vi "Subtract background.vi"(4 "Bin":dbl=0.05, 6 "Smoothing":dbl=32.0 format="%0.4f", 10 "Background":path=path "C:/Data/February_2015/021015/PDO_perp/s024_021015_TDO001.dat", 11 "Data":path=path "C:/Data/February_2015/021015/PDO_perp/s007_021015_TDO001.dat") -> (3 "XY Graph":cluster{"Output":dbl[], dbl[]}[](graph))   [LabVIEW 2018]
uses:
  <vilib>/Analysis/polynomials.llb/1D Polynomial Evaluation (DBL).vi
  <vilib>/Utility/file.llb/Write To Spreadsheet File (DBL).vi
  <vilib>/Analysis/NI_AALPro.lvlib
panel:
  in  "Keep old data":bool
  in  "Save result":bool=TRUE
  out "Waveform Graph":dbl[][](graph)
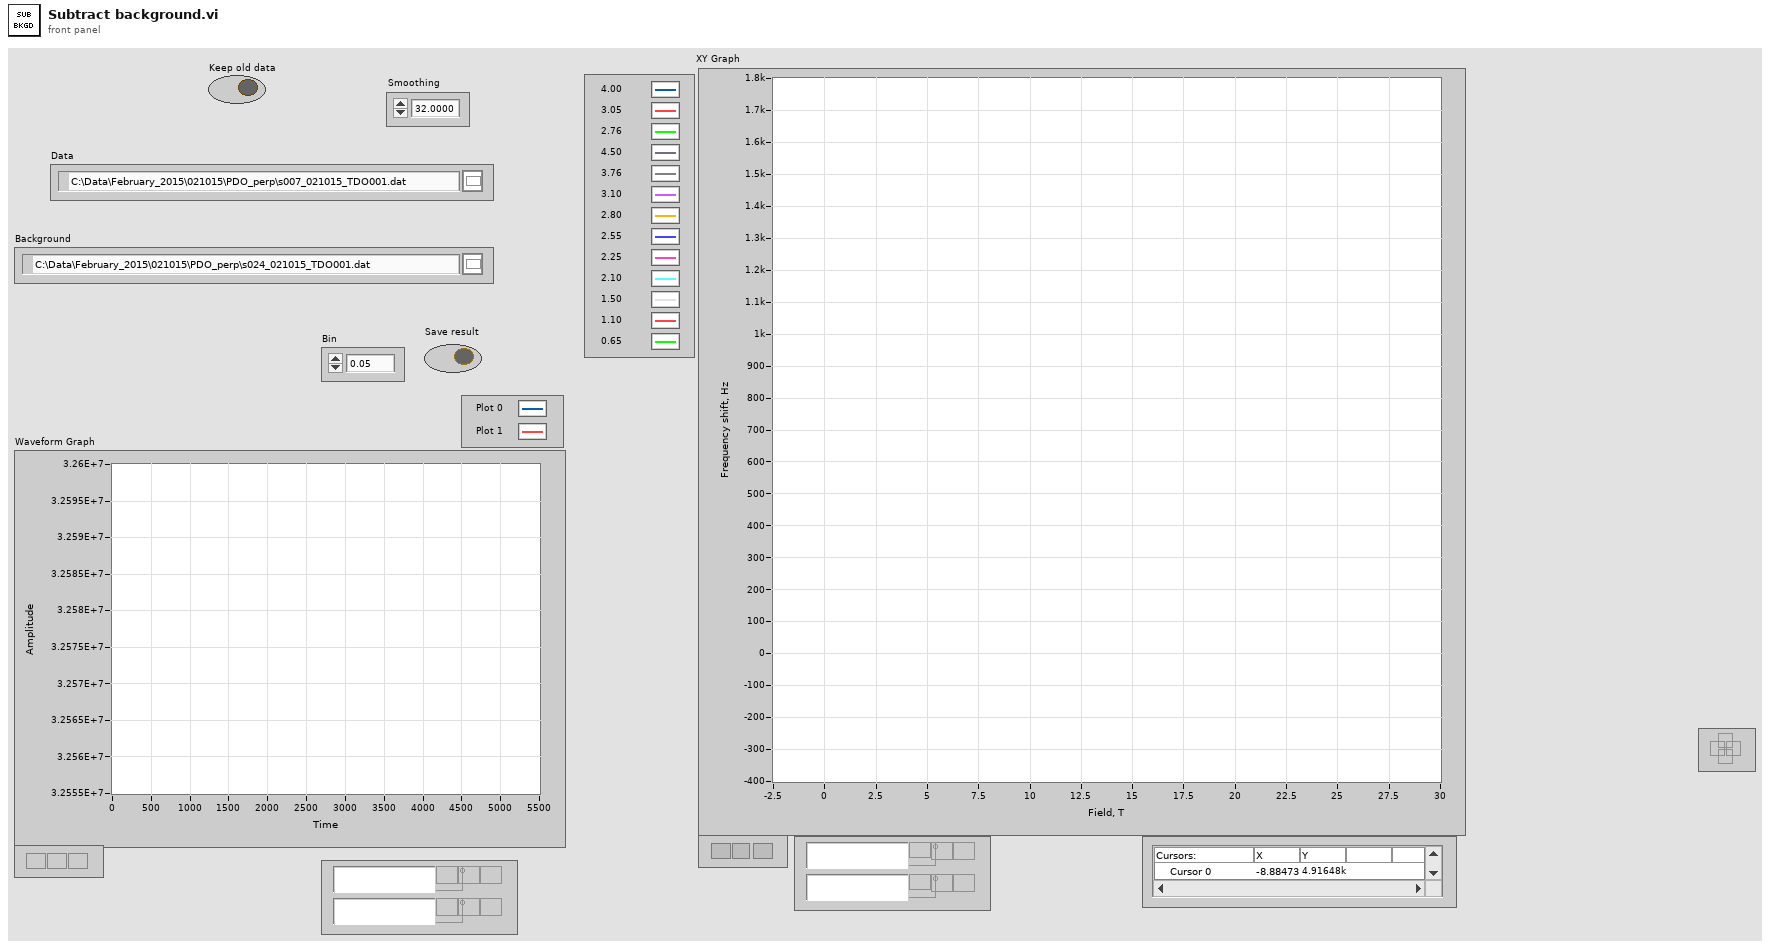
[diagram p1: front panel]
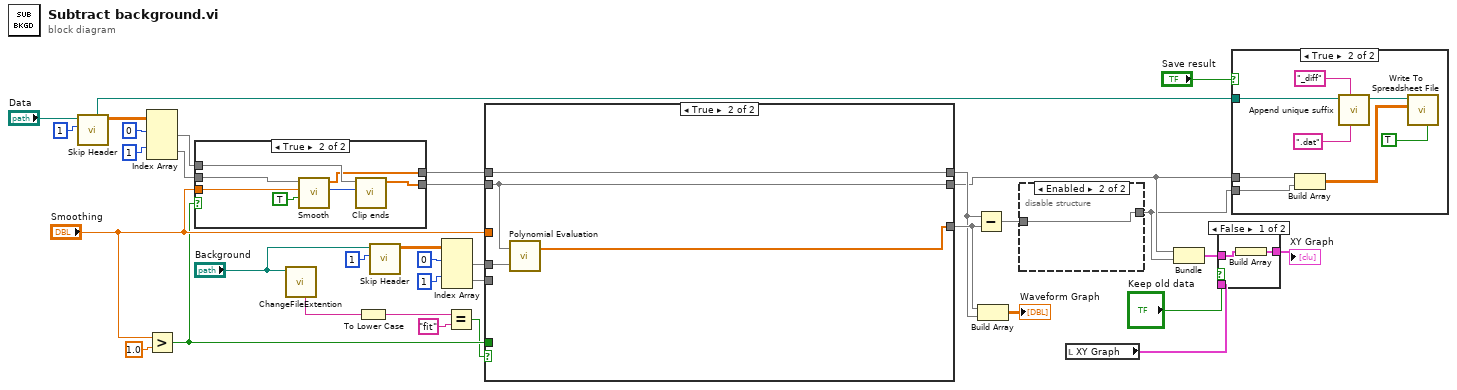
[diagram p0: block diagram]
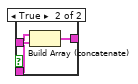
[diagram p2: hidden frame]
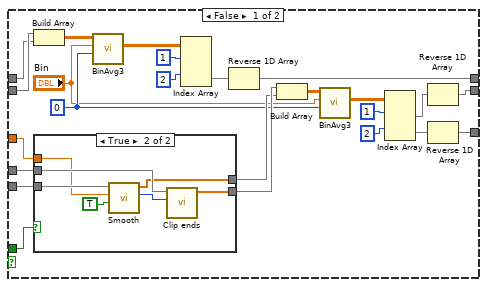
[diagram p3: hidden frame]
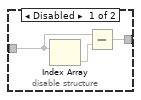
[diagram p6: hidden frame]
diagram:
  n1 = call "Skip Header.vi"("number of header lines"=1, "Input File Name"="Data") -> ("all rows"=w28:dbl[][], "new file path (Not A Path if cancelled)"=w12:path)  [unwired: 6 in, 2 out]
  n2 = Index Array(array=w28, index (row) #1=0 ("index (row)"), index (row) #2=1 ("index (row)")) -> (element #1=w24:dbl[], element #2=w25:dbl[])  [unwired: 2 in]
  n3 = Greater?(x="Smoothing", y=1.0) -> (0:w17:bool)
  n4 = case shown="True" w17 {
    tunnel: w25 -> [w37 w44]
    tunnel: [w37 w39] -> w21
    tunnel: "Smoothing" -> [_ w43]
    tunnel: w24 -> [w36 w41]
    tunnel: [w36 w38] -> w22
    frame False {
    }
    frame True {
      n5 = call "Smooth.vi"("Clip end ramps"=TRUE, "Smooth point width"=w43, "Input"=w44) -> ("Clip length"=w40:i32, "Output"=w39:dbl[])  [unwired: 7 in]
      n6 = call "Clip ends.vi"("Clip length"=w40, "Input"=w41) -> ("Output"=w38:dbl[])  [unwired: 9 in]
    }
  }
  n7 = call "ChangeFileExtention.vi"("Path"="Background") -> ("Old Extension"=w8:string)  [unwired: 6 in, 4 out]
  n8 = To Lower Case(string=w8) -> (all lower case string=w7:string)
  n9 = call "Skip Header.vi"("number of header lines"=1, "Input File Name"="Background") -> ("all rows"=w33:dbl[][])  [unwired: 6 in, 3 out]
  n10 = Index Array(array=w33, index (row) #1=0 ("index (row)"), index (row) #2=1 ("index (row)")) -> (element #1=w30:dbl[], element #2=w31:dbl[])  [unwired: 2 in]
  n11 = Equal?(x=w7, y="fit" ("Old Extension")) -> (x = y?=w5:bool)
  n12 = case shown="True" w5 {
    tunnel: w31 -> [w68 _]
    tunnel: w30 -> [w67 w81]
    tunnel: w22 -> [w60 w78]
    tunnel: w21 -> [w59 w80]
    tunnel: "Smoothing" -> [w50 _]
    tunnel: w17 -> [w49 _]
    tunnel: [w47 w79] -> w16
    tunnel: [w46 w80] -> w15
    tunnel: [w45 w78] -> w11
    frame False {
      w57 = 0 ("X coumn index")
      n13 = Build Array(w60, w59) -> (w58:dbl[][])
      n14 = case shown="True" w49 {
        tunnel: w68 -> [w70 w77]
        tunnel: [w70 w73] -> w62
        tunnel: w67 -> [w69 w75]
        tunnel: [w69 w72] -> w63
        tunnel: w50 -> [_ w71]
        frame False {
        }
        frame True {
          n15 = call "Smooth.vi"("Clip end ramps"=TRUE, "Smooth point width"=w71, "Input"=w77) -> ("Clip length"=w74:i32, "Output"=w73:dbl[])  [unwired: 7 in]
          n16 = call "Clip ends.vi"("Clip length"=w74, "Input"=w75) -> ("Output"=w72:dbl[])  [unwired: 9 in]
        }
      }
      n17 = call "BinAvg3.vi"("X coumn index"=w57, "Bin size"="Bin", "Data in"=w58) -> ("Binned data down"=w54:dbl[][])  [unwired: 1 in, 7 out]
      n18 = Index Array(array=w54, index (row) #1=1 ("index (row)"), index (row) #2=2 ("index (row)")) -> (element #2=w51:dbl[])  [unwired: 2 in, 1 out]
      n19 = Reverse 1D Array(array=w51) -> (reversed array=w46:dbl[])
      n20 = Build Array(w63, w62) -> (w61:dbl[][])
      n21 = call "BinAvg3.vi"("X coumn index"=w57, "Bin size"="Bin", "Data in"=w61) -> ("Binned data down"=w66:dbl[][])  [unwired: 1 in, 7 out]
      n22 = Index Array(array=w66, index (row) #1=1 ("index (row)"), index (row) #2=2 ("index (row)")) -> (element #1=w53:dbl[], element #2=w52:dbl[])  [unwired: 2 in]
      n23 = Reverse 1D Array(array=w53) -> (reversed array=w45:dbl[])
      n24 = Reverse 1D Array(array=w52) -> (reversed array=w47:dbl[])
    }
    frame True {
      n25 = call-poly <vilib>:"Polynomial Evaluation.vi"("P(x)"=w81, "A"=w78) -> ("P(A)"=w79:dbl[])  [unwired: 1 out]
    }
  }
  n26 = Subtract(x=w15, y=w16) -> (x-y=w14:dbl[])
  n27 = Build Array(w16, w15) -> (→"Waveform Graph":dbl[][])
  n28 = disable-structure shown="Enabled" {
    disable-tunnel: [w84 w85] -> w10
    disable-tunnel: w14 -> [w83 w85]
    frame Disabled {
      n29 = Index Array(array=w83) -> (element=w82:dbl)  [unwired: 1 in]
      n30 = Subtract(x=w83, y=w82) -> (x-y=w84:dbl[])
    }
    frame Enabled {
    }
  }
  n31 = local read "XY Graph"() -> (w2:cluster{"Output":dbl[], dbl[]}[])
  n32 = Bundle("Output"=w11, w10) -> (w4:cluster{"Output":dbl[], dbl[]})  [unwired: 1 in]
  n33 = case shown="False" "Keep old data" {
    tunnel: w4 -> [w87 w90]
    tunnel: [w86 w89] -> w3
    tunnel: w2 -> [_ w88]
    frame False {
      n34 = Build Array(w87) -> (w86:cluster{"Output":dbl[], dbl[]}[])
    }
    frame True {
      n35 = Build Array (concatenate)(w88, w90) -> (w89:cluster{"Output":dbl[], dbl[]}[])
    }
  }
  "XY Graph" <- w3
  n36 = case shown="True" "Save result" {
    tunnel: w12 -> [_ w96]
    tunnel: w11 -> [_ w94]
    tunnel: w10 -> [_ w93]
    frame False {
    }
    frame True {
      n37 = Build Array(w94, w93) -> (w92:dbl[][])
      n38 = call "Append unique suffix.vi"("Extention"=".dat", "Suffix"="_diff", "Path"=w96) -> ("Path out"=w95:path)  [unwired: 7 in, 1 out]
      n39 = call-poly <vilib>:"Write To Spreadsheet File.vi"("transpose? (no:F)"=TRUE, "2D data"=w92, "file path (dialog if empty)"=w95) -> ()  [unwired: 5 in, 1 out]
    }
  }
